vi "Load_RegData_Type.vi"(8 "error in (no error)":errorcluster, 9 "index in":string, 11 "buildObject":T1) -> (0 "error out":errorcluster, 1 "index out":string, 3 "IB_RegData out":refnum<class "IB_RegData.lvclass">)   [LabVIEW 2020, in "IB_RegData.lvclass"]
uses:
  <vilib>/AppBuilder/IB_Classes/RegData/IB_RegData.lvclass
  <vilib>/AppBuilder/IB_Classes/RegData/IB_RegData.lvclass/IB_RegData.ctl
  <vilib>/AppBuilder/IB_Classes/RegData/RegData_I32/IB_RegData_I32.lvclass
  <vilib>/AppBuilder/IB_Classes/RegData/RegData_String/IB_RegData_String.lvclass
  e:/builds/penguin/labview/branches/2020/dev/dist/vi.lib/AppBuilder/IB_Classes/RegData/IB_RegData.lvclass
  e:/builds/penguin/labview/branches/2020/dev/dist/vi.lib/AppBuilder/IB_Classes/RegData/RegData_I32/IB_RegData_I32.lvclass
  e:/builds/penguin/labview/branches/2020/dev/dist/vi.lib/AppBuilder/IB_Classes/RegData/RegData_String/IB_RegData_String.lvclass
  <resource>/Framework/Providers/API/ItemRef.ctl
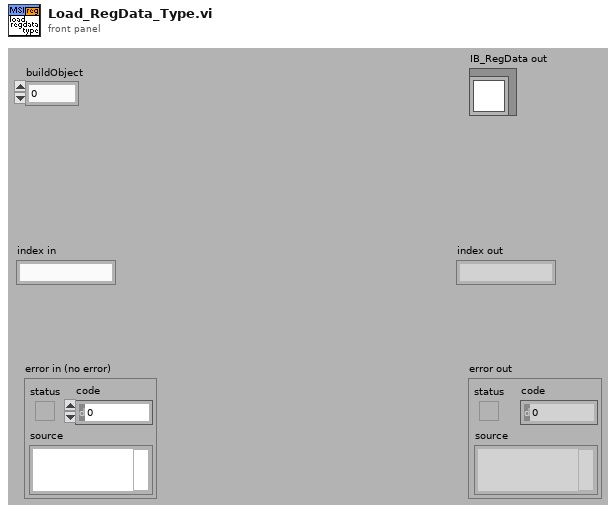
[diagram p1: front panel]
types:
  T1 = typedef "ItemRef.ctl" = u64
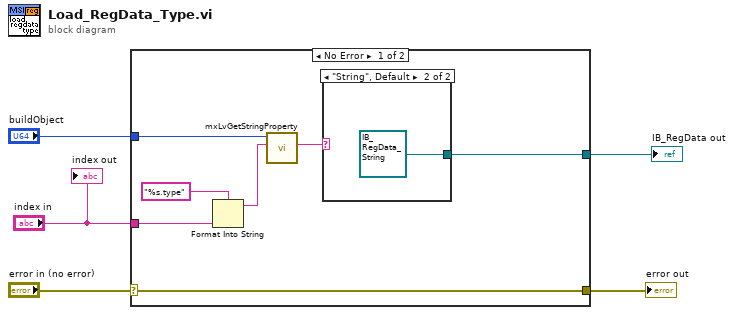
[diagram p0: block diagram]
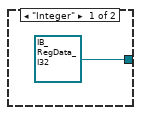
[diagram p2: hidden frame]
diagram:
  n1 = case shown="No Error" "error in (no error)" {
    selector: "error in (no error)" -> [w12 w15]
    tunnel: [w12 w15] -> w4
    tunnel: "index in" -> [w9 _]
    tunnel: "buildObject" -> [w8 _]
    tunnel: [w6 _] -> w1
    frame No Error {
      n2 = Format Into String(format string="%s.type", w9) -> (resulting string=w10:string)  [unwired: 2 in, 1 out]
      n3 = call <resource>:"mxLvGetStringProperty.vi"("Tag"=w10, "Item"=w8) -> ("Value"=w7:string)  [unwired: 1 in, 8 out]
      n4 = case shown="\"String\", Default" w7 {
        tunnel: [refnum<class "IB_RegData_I32.lvclass"> refnum ("IB_RegData_I32.lvclass") refnum<class "IB_RegData_String.lvclass"> refnum ("IB_RegData_String.lvclass")] -> w6
        frame "Integer" {
        }
        frame "String", Default {
        }
      }
    }
    frame Error {
    }
  }
  "error out" <- w4
  "IB_RegData out" <- w1
  "index out" <- "index in"
